vi "ListAllFolderRecursion.vi"(11 "Path":path=path "C:/Users/chrismadlax/Desktop/LVSampleCode/Recursion/testsample") -> (3 "PathArray":path[](array[path]))   [LabVIEW 2021]
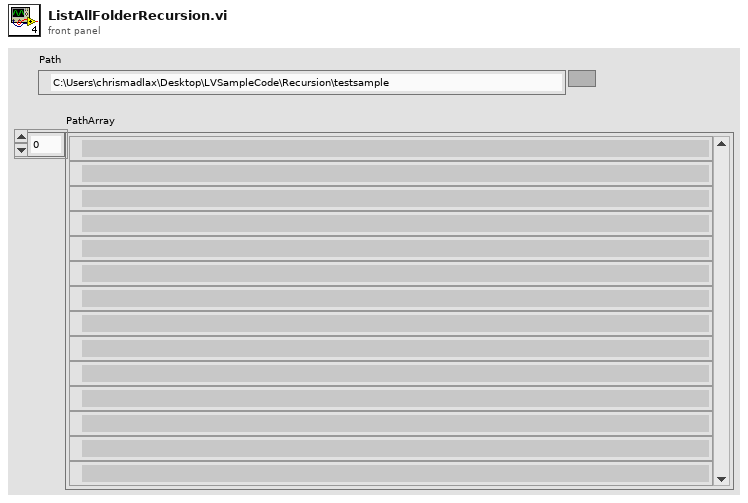
[diagram p1: front panel]
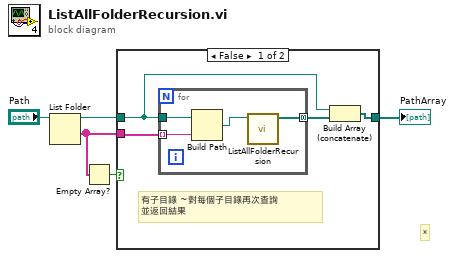
[diagram p0: block diagram]
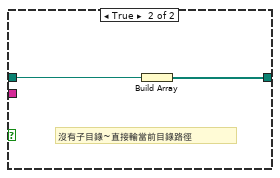
[diagram p2: hidden frame]
diagram:
  # "*"
  n1 = List Folder(path="Path") -> (path out=w4:path, folder names=w2:string[])  [unwired: 3 in, 2 out]
  n2 = Empty Array?(array=w2) -> (empty?=w3:bool)
  n3 = case shown="False" w3 {
    tunnel: w4 -> [w6 w15]
    tunnel: w2 -> [w8 _]
    tunnel: [w7 w14] -> w1
    frame False {
      # "有子目錄 ~對每個子目錄再次查詢\n並返回結果"
      n4 = for {
        tunnel: w6 -> [w13]
        tunnel: [w10] -> w9 mode=concatenating
        tunnel: w8 -> [w12] mode=indexing
        n5 = Build Path(base path=w13, name or relative path=w12) -> (appended path=w11:path)
        n6 = call "ListAllFolderRecursion.vi"("Path"=w11) -> ("PathArray"=w10:path[])  [unwired: 10 in]
      }
      n7 = Build Array (concatenate)(w6, w9) -> (w7:path[])
    }
    frame True {
      # "沒有子目錄~直接輸當前目錄路徑"
      n8 = Build Array(w15) -> (w14:path[])
    }
  }
  "PathArray" <- w1
